vi "Configure Branch Counter.vi"(7 "Target Count (0)":u32, 8 "error in (no error)":errorcluster, 9 "Branch To Block (0)":u32, 10 "Block Number (1)":u32=1, 11 "VISA resource name":refnum<visa-resource-name>) -> (0 "error out":errorcluster, 3 "VISA resource name out":refnum<visa-resource-name>)   [LabVIEW 2015, in "Keithley DMM6500 DAQ6500 Series.lvlib"]
doc: "Defines a trigger model block that branches to a specified block a specified number of times."
uses:
  <instrlib>/Keithley DMM6500 DAQ6500 Series/Keithley DMM6500 DAQ6500 Series.lvlib
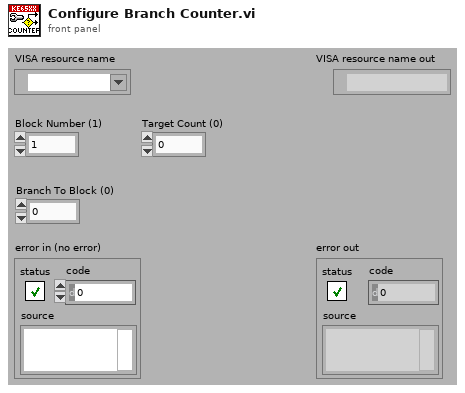
[diagram p1: front panel]
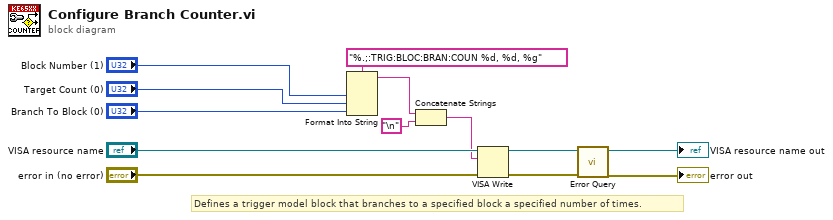
[diagram p0: block diagram]
diagram:
  # "Defines a trigger model block that branches to a specified block a specified number of times."
  n1 = Format Into String(format string="%.;:TRIG:BLOC:BRAN:COUN %d, %d, %g", "Block Number (1)", "Target Count (0)", "Branch To Block (0)") -> (resulting string=w2:string)  [unwired: 2 in, 1 out]
  n2 = Concatenate Strings(w2, "\n") -> (w3:string)
  n3 = VISA Write(VISA resource name="VISA resource name", write buffer=w3, error in (no error)="error in (no error)") -> (VISA resource name out=w7:refnum<visa-resource-name>, error out=w6:errorcluster)  [unwired: 1 out]
  n4 = call <instrlib>:"Error Query.vi"("error in (no error)"=w6, "VISA resource name"=w7) -> ("error out"=→"error out":errorcluster, "VISA resource name out"=→"VISA resource name out":refnum<visa-resource-name>)  [unwired: 6 in, 2 out]
